vi "SetWaitForTemp_popup.vi"(0 "VISA resource name":refnum<visa-resource-name>, 1 "Input Line Command":string, 2 "Condition":string(combo), 3 "error in (no error)":errorcluster, 4 "Timeout":string, 5 "Temperature":string, 6 "Sensor":string(combo), 7 "Controller":string(combo)) -> (8 "Output Line Command":string, 9 "Cancel":bool, 10 "error out":errorcluster)   [LabVIEW 2019]
panel:
  in  "platform":u16(ring) items=["Mac", "PC"]
  in  "Cancel button":bool
  in  "OK Button":bool
  # "K"
  # "(larger, smaller or close to (within 1%))"
  # "min"
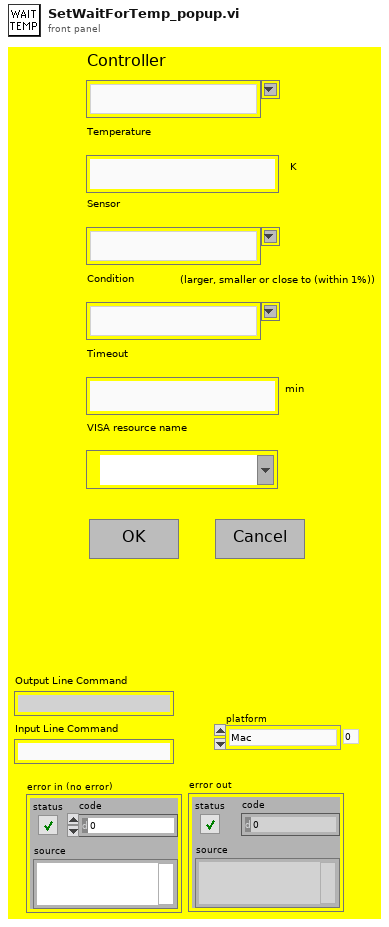
[diagram p1: front panel]
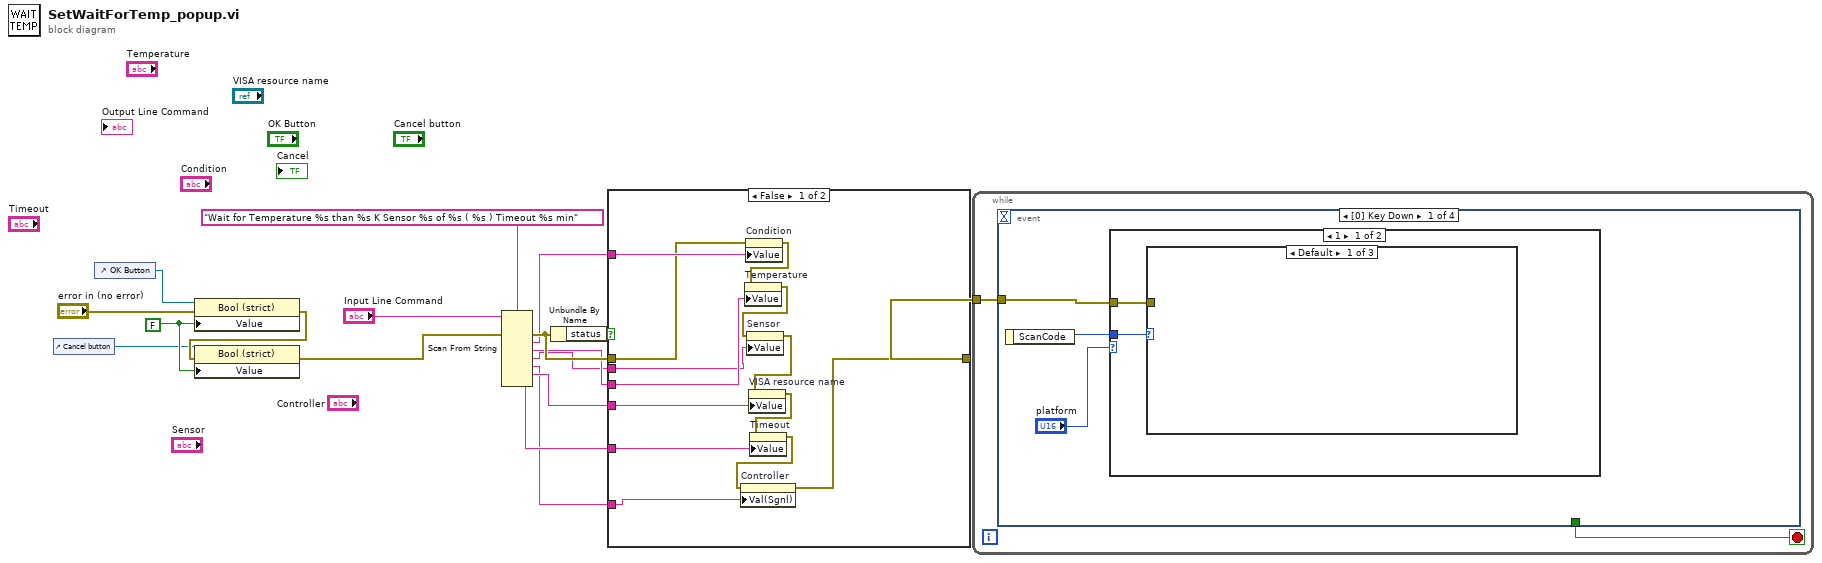
[diagram p0: block diagram]
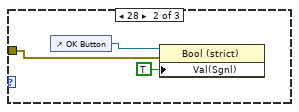
[diagram p2: hidden frame]
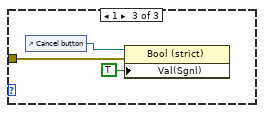
[diagram p3: hidden frame]
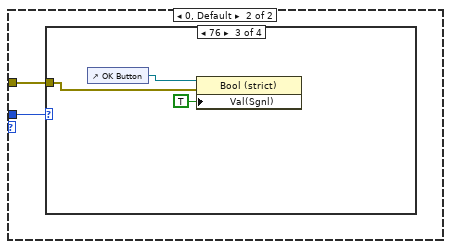
[diagram p4: hidden frame]
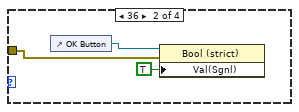
[diagram p6: hidden frame]
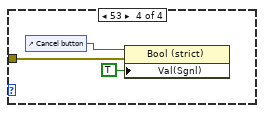
[diagram p7: hidden frame]
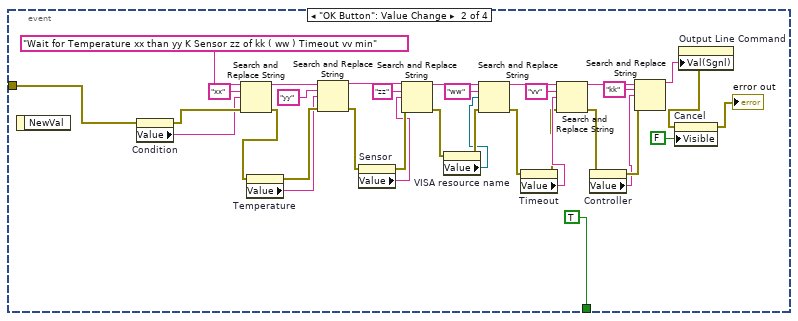
[diagram p8: hidden frame]
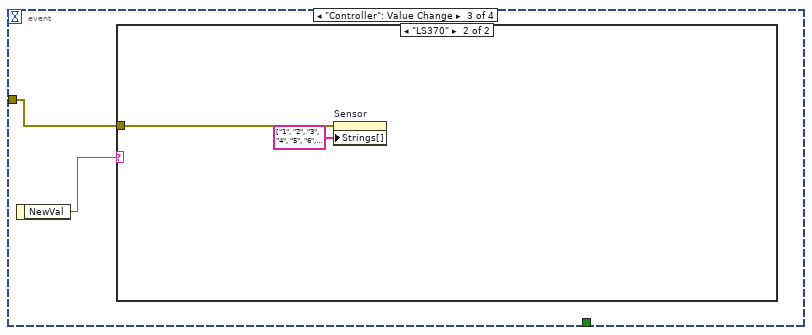
[diagram p9: hidden frame]
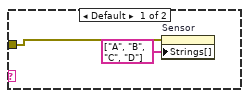
[diagram p10: hidden frame]
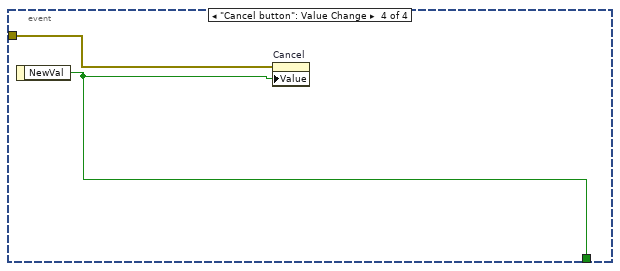
[diagram p11: hidden frame]
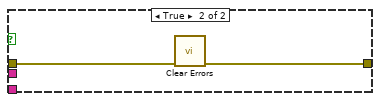
[diagram p12: hidden frame]
diagram:
  w16 = FALSE
  n1 = control-ref of="Cancel button"() -> (w13:refnum<vi>)
  n2 = control-ref of="OK Button"() -> (w14:refnum<vi>)
  n3 = property on="Property Node" class="Bool (strict)"(reference=w14, error in="error in (no error)", "Value"=w16) -> (error out=w15:errorcluster)  [unwired: 1 out]
  n4 = property on="Property Node" class="Bool (strict)"(reference=w13, error in=w15, "Value"=w16) -> (error out=w11:errorcluster)  [unwired: 1 out]
  n5 = Scan From String(format string="Wait for Temperature %s than %s K Sensor %s of %s ( %s ) Timeout %s min", input string="Input Line Command", error in=w11) -> (error out=w8:errorcluster, output 1=w7:string, output 2=w6:string, output 3=w5:string, output 4=w1:string, output 5=w2:string, output 6=w3:string)  [unwired: 7 in, 2 out]
  n6 = Unbundle By Name(w8) -> ("status"=w9:bool)
  n7 = case shown="False" w9 {
    tunnel: w8 -> [w29 w32]
    tunnel: [w19 w31] -> w4
    tunnel: w7 -> [w30 _]
    tunnel: w6 -> [w27 _]
    tunnel: w5 -> [w25 _]
    tunnel: w2 -> [w24 _]
    tunnel: w3 -> [w21 _]
    tunnel: w1 -> [w18 _]
    frame False {
      n8 = property on="Condition" class="CmbBox"(error in=w29, "Value"=w30) -> (error out=w28:errorcluster)  [unwired: 1 in, 1 out]
      n9 = property on="Temperature" class="Str"(error in=w28, "Value"=w27) -> (error out=w26:errorcluster)  [unwired: 1 in, 1 out]
      n10 = property on="Sensor" class="CmbBox"(error in=w26, "Value"=w25) -> (error out=w23:errorcluster)  [unwired: 1 in, 1 out]
      n11 = property on="VISA resource name" class="VISAName"(error in=w23, "Value"=w24) -> (error out=w22:errorcluster)  [unwired: 1 in, 1 out]
      n12 = property on="Timeout" class="Str"(error in=w22, "Value"=w21) -> (error out=w20:errorcluster)  [unwired: 1 in, 1 out]
      n13 = property on="Controller" class="CmbBox"(error in=w20, "Val(Sgnl)"=w18) -> (error out=w19:errorcluster)  [unwired: 1 in, 1 out]
    }
    frame True {
      n14 = call <vilib>:"Clear Errors.vi"("error in (no error)"=w32) -> ("error out"=w31:errorcluster)  [unwired: 5 in, 1 out]
    }
  }
  n15 = while {
    tunnel: w4 -> [w34]
    stop <- w33 stop-if-true
    n16 = event shown="[0] Key Down" {
      selector: _ -> [_ _ _ _]
      dyn-events: _ -> [_ _ _ _]
      timeout: _ -> [_ _ _ _]
      tunnel: w34 -> [w36 w89 w92 w99]
      tunnel: [_ TRUE _ w98] -> w33
      event Key Down {
        n17 = event-data() -> ("ScanCode"=w37:i16)  [unwired: 1 in]
        n18 = case shown="1" "platform" {
          tunnel: w37 -> [w39 w47]
          tunnel: w36 -> [w38 w46]
          frame 1 {
            n19 = case shown="Default" w39 {
              tunnel: w38 -> [_ w41 w44]
              frame Default {
              }
              frame 28 {
                n20 = control-ref of="OK Button"() -> (w42:refnum<vi>)
                n21 = property on="Property Node" class="Bool (strict)"(reference=w42, error in=w41, "Val(Sgnl)"=TRUE ("Value (Signaling)")) -> ()  [unwired: 2 out]
              }
              frame 1 {
                n22 = control-ref of="Cancel button"() -> (w45:refnum<vi>)
                n23 = property on="Property Node" class="Bool (strict)"(reference=w45, error in=w44, "Val(Sgnl)"=TRUE ("Value (Signaling)")) -> ()  [unwired: 2 out]
              }
            }
          }
          frame 0, Default {
            n24 = case shown="76" w47 {
              tunnel: w46 -> [_ w49 w52 w55]
              frame Default {
              }
              frame 36 {
                n25 = control-ref of="OK Button"() -> (w50:refnum<vi>)
                n26 = property on="Property Node" class="Bool (strict)"(reference=w50, error in=w49, "Val(Sgnl)"=TRUE ("Value (Signaling)")) -> ()  [unwired: 2 out]
              }
              frame 76 {
                n27 = control-ref of="OK Button"() -> (w53:refnum<vi>)
                n28 = property on="Property Node" class="Bool (strict)"(reference=w53, error in=w52, "Val(Sgnl)"=TRUE ("Value (Signaling)")) -> ()  [unwired: 2 out]
              }
              frame 53 {
                n29 = control-ref of="Cancel button"() -> (w56:refnum<vi>)
                n30 = property on="Property Node" class="Bool (strict)"(reference=w56, error in=w55, "Val(Sgnl)"=TRUE ("Value (Signaling)")) -> ()  [unwired: 2 out]
              }
            }
          }
        }
      }
      event "OK Button": Value Change {
        n31 = event-data() -> ()  [unwired: 1 in, 1 out]
        n32 = property on="Condition" class="CmbBox"(error in=w89) -> (error out=w88:errorcluster, "Value"=w87:string)  [unwired: 1 in, 1 out]
        n33 = Search and Replace String(input string="Wait for Temperature xx than yy K Sensor zz of kk ( ww ) Timeout vv min" ("format string"), search string="xx", replace string=w87, error in=w88) -> (result string=w86:string, error out=w84:errorcluster)  [unwired: 4 in, 2 out]
        n34 = property on="Temperature" class="Str"(error in=w84) -> (error out=w83:errorcluster, "Value"=w82:string)  [unwired: 1 in, 1 out]
        n35 = Search and Replace String(input string=w86, search string="yy", replace string=w82, error in=w83) -> (result string=w81:string, error out=w78:errorcluster)  [unwired: 4 in, 2 out]
        n36 = property on="Sensor" class="CmbBox"(error in=w78) -> (error out=w77:errorcluster, "Value"=w76:string)  [unwired: 1 in, 1 out]
        n37 = Search and Replace String(input string=w81, search string="zz", replace string=w76, error in=w77) -> (result string=w75:string, error out=w73:errorcluster)  [unwired: 4 in, 2 out]
        n38 = property on="VISA resource name" class="VISAName"(error in=w73) -> (error out=w72:errorcluster, "Value"=w71:refnum<visa-resource-name>)  [unwired: 1 in, 1 out]
        n39 = Search and Replace String(input string=w75, search string="ww", replace string=w71, error in=w72) -> (result string=w70:string, error out=w68:errorcluster)  [unwired: 4 in, 2 out]
        n40 = property on="Timeout" class="Str"(error in=w68) -> (error out=w66:errorcluster, "Value"=w67:string)  [unwired: 1 in, 1 out]
        n41 = Search and Replace String(input string=w70, search string="vv", replace string=w67, error in=w66) -> (result string=w62:string, error out=w59:errorcluster)  [unwired: 4 in, 2 out]
        n42 = property on="Controller" class="CmbBox"(error in=w59) -> (error out=w58:errorcluster, "Value"=w57:string)  [unwired: 1 in, 1 out]
        n43 = Search and Replace String(input string=w62, search string="kk", replace string=w57, error in=w58) -> (result string=w61:string)  [unwired: 4 in, 3 out]
        n44 = property on="Output Line Command" class="Str"("Val(Sgnl)"=w61) -> (error out=w65:errorcluster)  [unwired: 2 in, 1 out]
        n45 = property on="Cancel" class="Bool (strict)"(error in=w65, "Visible"=FALSE) -> (error out=→"error out":errorcluster)  [unwired: 1 in, 1 out]
      }
      event "Controller": Value Change {
        n46 = event-data() -> ("NewVal"=w93:string)  [unwired: 1 in]
        n47 = case shown="\"LS370\"" w93 {
          tunnel: w92 -> [w95 w97]
          frame Default {
            n48 = property on="Sensor" class="CmbBox"(error in=w95, "Strings[]"=string[] ["A", "B", "C", "D"] ("Strings []")) -> ()  [unwired: 1 in, 2 out]
          }
          frame "LS370" {
            n49 = property on="Sensor" class="CmbBox"(error in=w97, "Strings[]"=string[] ["1", "2", "3", "4", "5", "6", "7"] ("Strings []")) -> ()  [unwired: 1 in, 2 out]
          }
        }
      }
      event "Cancel button": Value Change {
        n50 = event-data() -> ("NewVal"=w98:bool)  [unwired: 1 in]
        n51 = property on="Cancel" class="Bool (strict)"(error in=w99, "Value"=w98) -> ()  [unwired: 1 in, 2 out]
      }
    }
  }
